vi "Read.vi"(0 "reference in":refnum<class "Barcode_Reader_Base.lvclass">, 5 "error in (no error)":errorcluster) -> (14 "reference in":refnum<class "Barcode_Reader_Base.lvclass">, 16 "Serial":string, 17 "read Ok":bool, 19 "error out":errorcluster)   [LabVIEW 2022 SP3, in "Barcode_Reader_Base.lvlib" / "Barcode_Reader_Base.lvclass"]
uses:
  Barcode_Reader_Base.lvclass
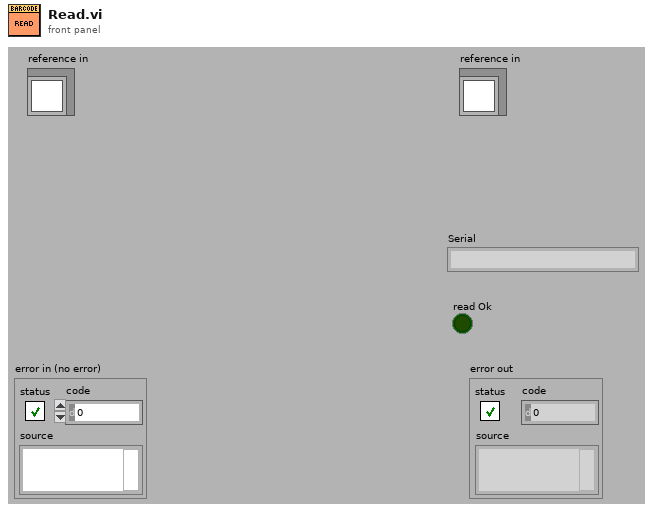
[diagram p1: front panel]
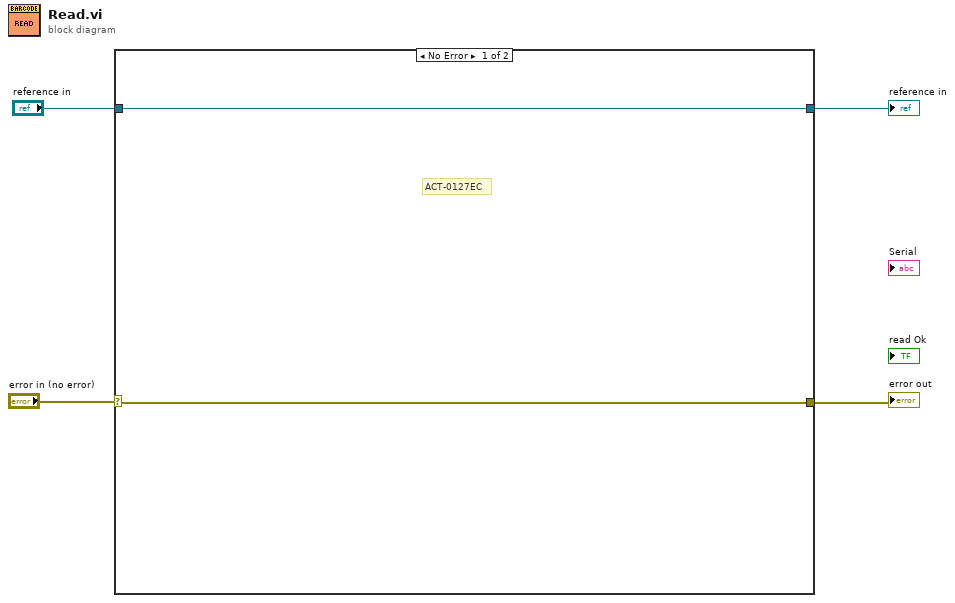
[diagram p0: block diagram]
diagram:
  n1 = case shown="No Error" "error in (no error)" {
    selector: "error in (no error)" -> [w5 w8]
    tunnel: [w5 w8] -> w3
    tunnel: [w6 w7] -> w1
    tunnel: "reference in" -> [w6 w7]
    frame No Error {
      # "ACT-0127EC"
    }
    frame Error {
    }
  }
  "error out" <- w3
  "reference in" <- w1
